vi "Path Finder.vi"(0 "Paths in":T2, 1 "Allowed Directions to move":T1[](array[typedef]), 2 "Destination Location":cdb, 3 "Current Location":cdb, 4 "Elevation Grid Numeric":i32[][](array[numeric]), 5 "Max Distance per step":cdb, 6 "Max Elevation per step":i32) -> (7 "Paths out":T2, 10 "Path available ?":bool)   [LabVIEW 2020, in "AoC 2022.lvlib"]
uses:
  AoC 2022.lvlib
  Paths.ctl
  Path.ctl
  Direction.ctl
  <vilib>/Utility/miscctls.llb/LVMapReplaceAction.ctl
  c269ea1d-287c-46b8-ae72-11cd65caee4e.vi
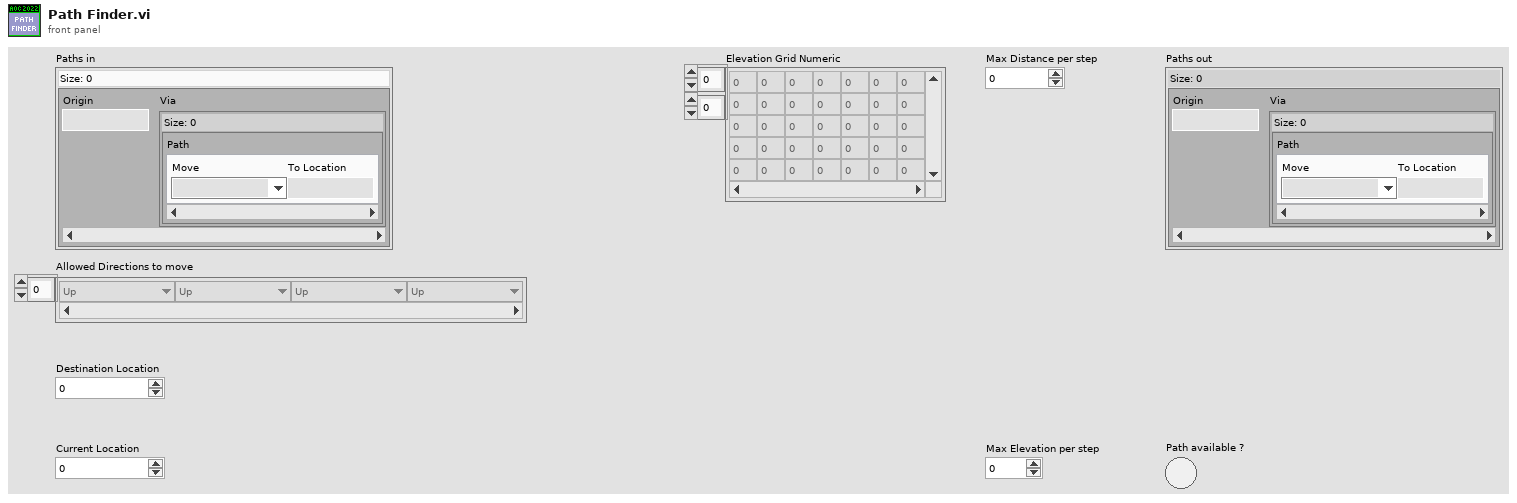
[diagram p1: front panel]
types:
  T1 = typedef "AoC 2022.lvlib/Direction.ctl" = enum16{"Up", "UpRight", "Right", "DownRight", "Down", "DownLeft", "Left", "UpLeft", "Stay"}
  T2 = typedef "AoC 2022.lvlib/Paths.ctl" = map{cdb, set{T3}}
  T3 = typedef "AoC 2022.lvlib/Path.ctl" = cluster{"Move":T1, "To Location":cdb}
  T4 = typedef "LVMapReplaceAction.ctl" = enum32{"Modify Entry only if found", "Add or Modify Entry", "Delete Entry"}
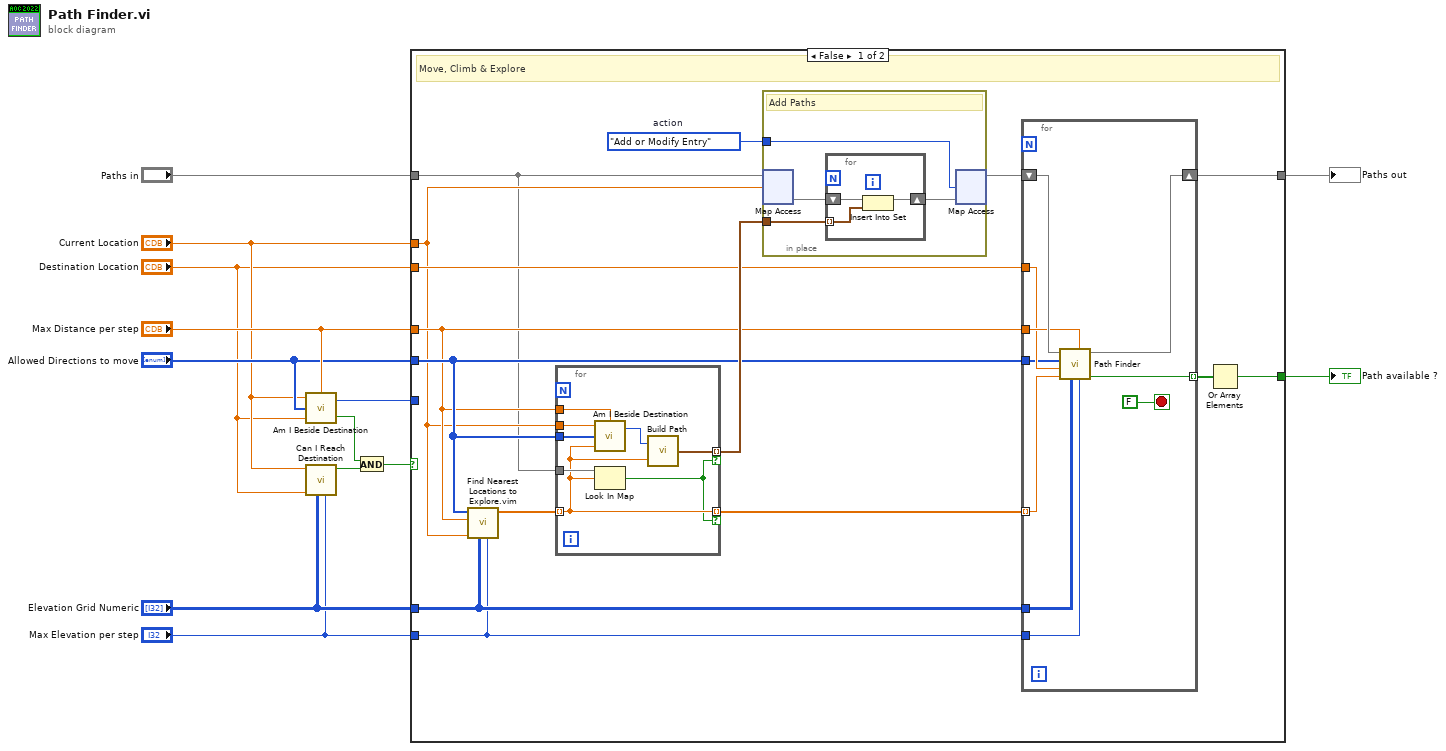
[diagram p0: block diagram]
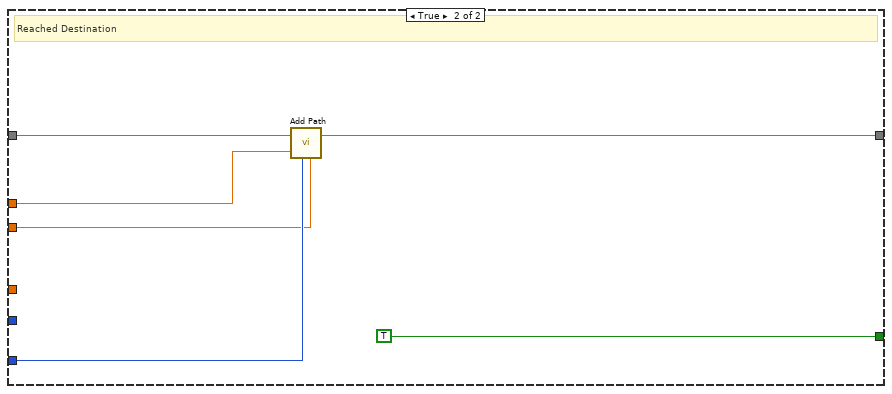
[diagram p2: hidden frame]
diagram:
  n1 = call "Am I Beside Destination.vi"("Max Distance per step"="Max Distance per step", "Destination Location"="Destination Location", "Allowed Directions to move"="Allowed Directions to move", "Current Location"="Current Location") -> ("Am I beside Destination ?"=w6:bool, "Direction to Destination"=w4:T1)
  n2 = call "Can I Reach Destination.vi"("Max Elevation per step"="Max Elevation per step", "Elevation Grid Numeric"="Elevation Grid Numeric", "Destination Location"="Destination Location", "Current Location"="Current Location") -> ("Can I reach Destination ?"=w3:bool)  [unwired: 5 in]
  n3 = And(x=w6, y=w3) -> (x .and. y?=w5:bool)
  n4 = case shown="False" w5 {
    tunnel: "Current Location" -> [w20 w58]
    tunnel: "Destination Location" -> [w25 w55]
    tunnel: w4 -> [_ w56]
    tunnel: [w26 w57] -> w12
    tunnel: "Paths in" -> [w16 w59]
    tunnel: [w18 TRUE] -> w13
    tunnel: "Max Distance per step" -> [w21 _]
    tunnel: "Elevation Grid Numeric" -> [w24 _]
    tunnel: "Max Elevation per step" -> [w23 _]
    tunnel: "Allowed Directions to move" -> [w22 _]
    frame False {
      w14 = LVMapReplaceAction."Add or Modify Entry"  # action
      # "Move, Climb & Explore"
      n5 = call "Find Nearest Locations to Explore.vim"("Max Elevation per step"=w23, "Elevation Grid Numeric"=w24, "Current Location"=w20, "Max Distance per step"=w21, "Allowed Directions to move"=w22) -> ("Nearest Locations to Explore"=w17:cdb[])  [unwired: 4 in]
      n6 = for {
        tunnel: w17 -> [w30] mode=indexing
        tunnel: w21 -> [w36]
        tunnel: w20 -> [w35]
        tunnel: [w33] -> w28 mode=indexing if=w29
        tunnel: w22 -> [w32]
        tunnel: w16 -> [w31]
        tunnel: [w30] -> w15 mode=indexing if=w29
        n7 = call "Am I Beside Destination.vi"("Max Distance per step"=w36, "Destination Location"=w30, "Allowed Directions to move"=w32, "Current Location"=w35) -> ("Direction to Destination"=w34:T1)  [unwired: 1 out]
        n8 = Look In Map(map=w31, key=w30) -> (key not found?=w29:bool)  [unwired: 1 in, 1 out]
        n9 = call "Build Path.vi"("To Location"=w30, "Move"=w34) -> ("Path"=w33:T3)
      }
      n10 = in-place {
        in-place-border: w28 -> [w48]
        in-place-border: w14 -> [w47]
        # "Add Paths"
        n11 = in-place-map #1(w16, w20) -> (w50:set{T3})  [unwired: 1 in, 1 out]
        n12 = for {
          tunnel: w48 -> [w51] mode=indexing
          shift-right: [w52] -> w49
          shift-left: w50 -> [w53]
          n13 = Insert Into Set(10:w51, 11:w53) -> (3:w52:set{T3})  [unwired: 1 out]
        }
        n14 = in-place-map #1(w49, w47) -> (w27:T2)  [unwired: 2 out]
      }
      n15 = for {
        tunnel: w24 -> [w46]
        tunnel: w23 -> [w45]
        shift-right: [w43] -> w26
        shift-left: w27 -> [w44]
        tunnel: w25 -> [w41]
        tunnel: w21 -> [w42]
        tunnel: w15 -> [w40] mode=indexing
        tunnel: w22 -> [w39]
        tunnel: [w38] -> w19 mode=indexing
        stop <- FALSE stop-if-true
        n16 = call "Path Finder.vi"("Paths in"=w44, "Allowed Directions to move"=w39, "Destination Location"=w41, "Current Location"=w40, "Elevation Grid Numeric"=w46, "Max Distance per step"=w42, "Max Elevation per step"=w45) -> ("Paths out"=w43:T2, "Path available ?"=w38:bool)  [unwired: 2 in]
      }
      n17 = Or Array Elements(Boolean array=w19) -> (logical OR=w18:bool)
    }
    frame True {
      # "Reached Destination"
      n18 = call "Add Path.vi"("Origin"=w58, "Move"=w56, "To Location"=w55, "Paths in"=w59) -> ("Paths out"=w57:T2)  [unwired: 3 in]
    }
  }
  "Path available ?" <- w13
  "Paths out" <- w12
